vi "SDR_FrConf.vi"(10 "UpDw_Ch":enum16{"Up_Rx", "Down_Tx"}(ring), 11 "RxFrequency":u32) -> (3 "string":string)   [LabVIEW 2015]
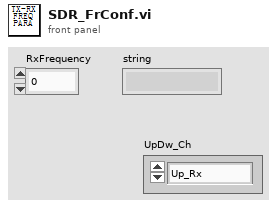
[diagram p1: front panel]
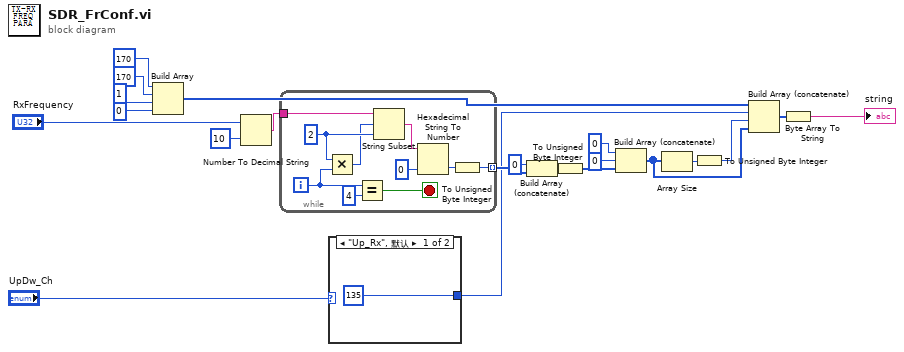
[diagram p0: block diagram]
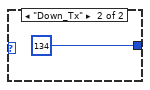
[diagram p2: hidden frame]
diagram:
  n1 = Build Array(u8 170, u8 170, u8 1, u8 0) -> (w20:u8[])
  n2 = Number To Decimal String(number="RxFrequency", width (-)=i16 10 ("宽度(-)")) -> (decimal integer string=w19:string)
  n3 = while {
    tunnel: w19 -> [w29]
    tunnel: [w22] -> w4 mode=indexing
    i -> [w27]
    stop <- w30 stop-if-true
    w28 = 2 ("长度（剩余）")
    n4 = Multiply(x=w28, y=w27) -> (x*y=w26:i32)
    n5 = Equal?(x=w27, y=4) -> (x = y?=w30:bool)
    n6 = String Subset(string=w29, offset (0)=w26, length (rest)=w28) -> (substring=w24:string)
    n7 = Hexadecimal String To Number(string=w24, default (0uL)=u8 0 ("默认(0 U32)")) -> (number=w23:u8)  [unwired: 2 out]
    n8 = To Unsigned Byte Integer(number=w23) -> (unsigned 8bit integer=w22:u8)
  }
  n9 = case shown="\"Up_Rx\", 默认" "UpDw_Ch" {
    tunnel: [u8 135 u8 134] -> w1
    frame "Up_Rx", Default {
    }
    frame "Down_Tx" {
    }
  }
  n10 = Build Array (concatenate)(u8 0 ("射频类型"), w4) -> (w5:u8[])
  n11 = To Unsigned Byte Integer(number=w5) -> (unsigned 8bit integer=w7:u8[])
  n12 = Build Array (concatenate)(u8 0, u8 0, w7) -> (w16:u8[])
  n13 = Array Size(array=w16) -> (size(s)=w14:i32)
  n14 = To Unsigned Byte Integer(number=w14) -> (unsigned 8bit integer=w15:u8)
  n15 = Build Array (concatenate)(w20, w1, w15, w16) -> (w17:u8[])
  n16 = Byte Array To String(unsigned byte array=w17) -> (string=→"string":string)
